vi "TimeEst to TimeDateStamp.vi"(8 "year":i32=1970, 9 "month":i32=1, 10 "day of month":i32=1, 11 "Time String":string) -> (3 "time stamp":timestamp)   [LabVIEW 2012]
uses:
  <vilib>/Utility/miscctls.llb/LVDateTimeRec.ctl
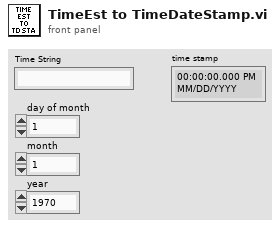
[diagram p1: front panel]
types:
  T1 = typedef "LVDateTimeRec.ctl" = cluster{"fractional second":dbl, "second":i32, "minute":i32, "hour":i32, "day of month":i32, "month":i32, "year":i32, "day of week":i32, "day of year":i32, "DST":i32}
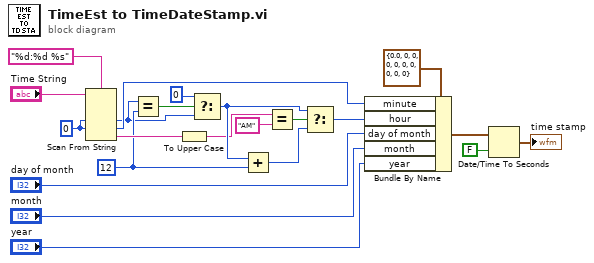
[diagram p0: block diagram]
diagram:
  w7 = 12 ("y")
  w20 = 0 ("default value 1")
  n1 = Scan From String(format string="%d:%d %s", input string="Time String", default 1=w20, default 2=w20) -> (output 1=w3:i32, output 2=w16:i32, output 3=w19:string)  [unwired: 3 in, 3 out]
  n2 = Equal?(x=w3, y=w7) -> (x = y?=w6:bool)
  n3 = To Upper Case(1:w19) -> (0:w2:string)
  n4 = Select(t=0, s=w6, f=w3) -> (s? t:f=w5:i32)
  n5 = Add(x=w5, y=w7) -> (x+y=w9:i32)
  n6 = Equal?(x=w2, y="AM") -> (x = y?=w8:bool)
  n7 = Select(t=w5, s=w8, f=w9) -> (s? t:f=w1:i32)
  n8 = Bundle By Name(cluster=T1 {"fractional second"=0.0, "second"=0, "minute"=0, "hour"=0, "day of month"=0, "month"=0, "year"=0, "day of week"=0, "day of year"=0, "DST"=0} ("date time rec"), "minute"=w16, "hour"=w1, "day of month"="day of month", "month"="month", "year"="year") -> (w17:T1)
  n9 = Date/Time To Seconds(1:FALSE ("is UTC (F)"), 2:w17) -> (0:→"time stamp":timestamp)
